vi "UDP_Basic_Client.vi"(4 "error In":errorcluster, 5 "Service Name":string, 6 "IP Adress":string, 7 "DataTypeIn":variant) -> (0 "error IO":errorcluster, 1 "String":string, 3 "DataOut":variant)   [LabVIEW 2010]
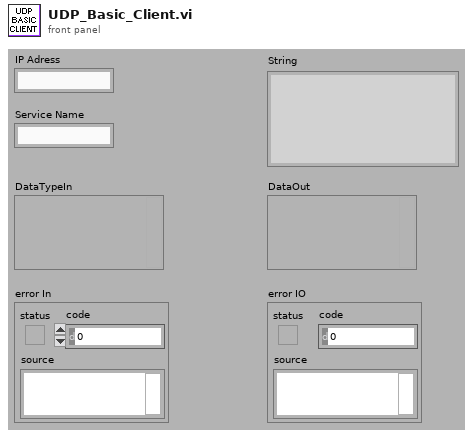
[diagram p1: front panel]
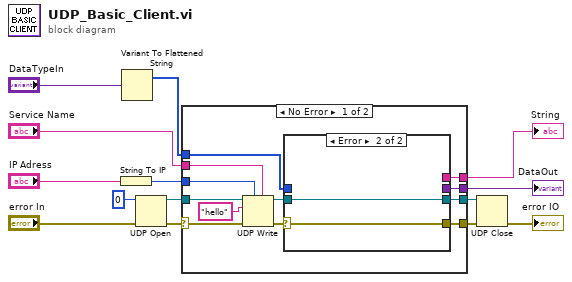
[diagram p0: block diagram]
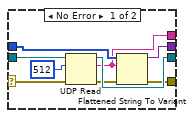
[diagram p2: hidden frame]
diagram:
  n1 = String To IP(1:"IP Adress") -> (0:w11:u32)
  n2 = Variant To Flattened String(Variant="DataTypeIn") -> (1:w13:i16[])  [unwired: 1 out]
  n3 = UDP Open(8:"error In", 11:u16 0 ("port")) -> (port=w7:refnum<k16>, 0:w8:errorcluster)  [unwired: 3 in, 1 out]
  n4 = case shown="No Error" w8 {
    selector: w8 -> [w26 w39]
    tunnel: [w15 w39] -> w1
    tunnel: w7 -> [w25 w38]
    tunnel: w13 -> [w22 _]
    tunnel: "Service Name" -> [w21 _]
    tunnel: w11 -> [w20 _]
    tunnel: [w19 _] -> w5
    tunnel: [w18 _] -> w4
    tunnel: [w16 w38] -> w2
    frame No Error {
      n5 = UDP Write(address=w20, port or service name=w21, connection ID=w25, data in="hello", 8:w26) -> (error out=w24:errorcluster, 3:w23:refnum<k16>)  [unwired: 1 in]
      n6 = case shown="Error" w24 {
        selector: w24 -> [w35 w36]
        tunnel: w23 -> [w34 w37]
        tunnel: [w32 w37] -> w16
        tunnel: [w28 w36] -> w15
        tunnel: w22 -> [w31 _]
        tunnel: [w29 _] -> w19
        tunnel: [w27 _] -> w18
        frame No Error {
          n7 = UDP Read(connection ID=w34, max size (548)=512, 8:w35) -> (data out=w27:string, error out=w30:errorcluster, 3:w32:refnum<k16>)  [unwired: 1 in, 2 out]
          n8 = Flattened String To Variant(4:w30, 6:w27, 7:w31) -> (0:w28:errorcluster, 3:w29:variant)
        }
        frame Error {
        }
      }
    }
    frame Error {
    }
  }
  "DataOut" <- w5
  "String" <- w4
  n9 = UDP Close(connection ID=w2, 8:w1) -> (error out=→"error IO":errorcluster)  [unwired: 1 out]
